vi "int16 to Hex.vi"(11 "number":dbl) -> (3 "Hex string":string)   [LabVIEW 2017]
panel:
  out "hex integer string":string
  # "RE-ENTRANT"
  # "SUB-ROUTINE"
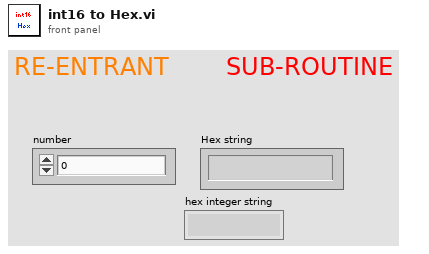
[diagram p1: front panel]
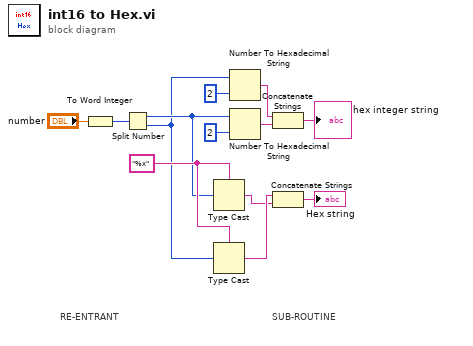
[diagram p0: block diagram]
diagram:
  w7 = "%x" ("type")
  # "SUB-ROUTINE"
  # "RE-ENTRANT"
  n1 = To Word Integer(number="number") -> (16bit integer=w11:i16)
  n2 = Split Number(x=w11) -> (hi(x)=w4:u8, lo(x)=w3:u8)
  n3 = Type Cast(type=w7, x=w4) -> (*(type *) &x=w1:string)
  n4 = Type Cast(type=w7, x=w3) -> (*(type *) &x=w2:string)
  n5 = Number To Hexadecimal String(1:i16 2 ("width (-)"), 2:w3) -> (0:w13:string)
  n6 = Number To Hexadecimal String(1:i16 2 ("width (-)"), 2:w4) -> (0:w12:string)
  n7 = Concatenate Strings(w13, w12) -> (→"hex integer string":string)
  n8 = Concatenate Strings(w2, w1) -> (→"Hex string":string)
